vi "Create from TCP-IP.vi"(5 "Local Host":string="127.0.0.1", 7 "Local Port":i32=2222, 8 "Error In":errorcluster, 9 "Remote Port":i32=22, 10 "Remote Host":string="127.0.0.1", 11 "Session":refnum<class "Session.lvclass">) -> (0 "Error Out":errorcluster, 3 "Channel":refnum<class "Channel.lvclass">)   [LabVIEW 2018, in "Toolkit.lvlib" / "Channel.lvclass"]
uses:
  Channel.lvclass
  Session/Session.lvclass
  Session/Session.lvclass/Session.ctl
  SSH/SSH.lvclass/SSH.ctl
  Channel.lvclass/Channel.ctl
  Toolkit.lvlib
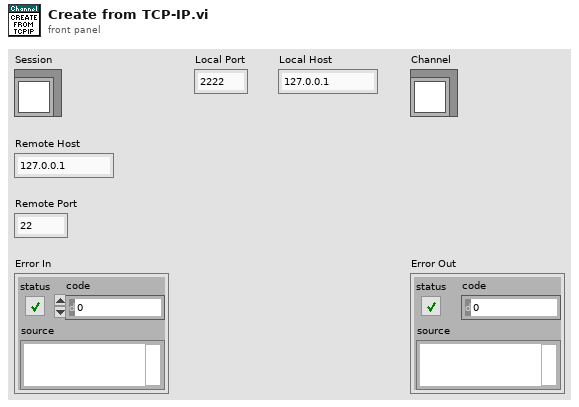
[diagram p1: front panel]
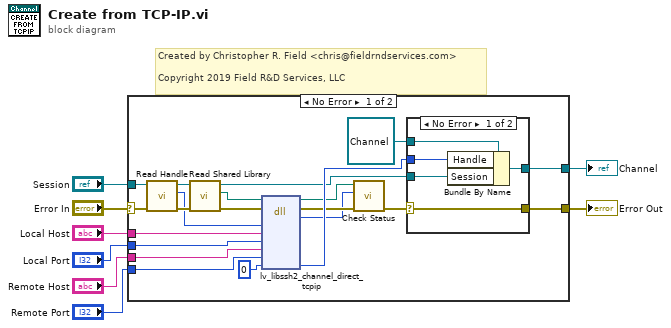
[diagram p0: block diagram]
diagram:
  # "Created by Christopher R. Field <chris@fieldrndservices.com>\n\nCopyright 2019 Field R&D Services, LLC"
  n1 = case shown="No Error" "Error In" {
    selector: "Error In" -> [w27 w37]
    tunnel: [w15 w37] -> w7
    tunnel: "Session" -> [w28 _]
    tunnel: [w29 _] -> w5
    tunnel: "Local Host" -> [w12 _]
    tunnel: "Local Port" -> [w11 _]
    tunnel: "Remote Host" -> [w10 _]
    tunnel: "Remote Port" -> [w9 _]
    frame No Error {
      n2 = call "Read Handle.vi"("Error In"=w27, "Session In"=w28) -> ("Erorr Out"=w25:errorcluster, "Handle"=w22:u64, "Session Out"=w26:refnum<class "Session.lvclass">)  [unwired: 7 in]
      n3 = call "Read Shared Library.vi"("Error In"=w25, "Session In"=w26) -> ("Erorr Out"=w24:errorcluster, "libssh2lv Shared Library"=w23:path, "Session Out"=w14:refnum<class "Session.lvclass">)  [unwired: 7 in]
      n4 = dll-call lib="libssh2lv.*" fn="lv_libssh2_channel_direct_tcpip"(path in=w23, error in=w24, "session"=w22, "host"=w12, "port"=w11, "server_host"=w10, "server_port"=w9, "handle"=u64 0) -> (path out=w17:path, error out=w19:errorcluster, "status"=w18:i32, "handle"=w20:u64)  [unwired: 6 in]
      n5 = call "Check Status.vi"("Error In"=w19, "Status"=w18, "lv-libssh2 Shared Library In"=w17) -> ("Error Out"=w16:errorcluster)  [unwired: 7 in, 1 out]
      n6 = case shown="No Error" w16 {
        selector: w16 -> [w33 w36]
        tunnel: [w30 w35] -> w29
        tunnel: w20 -> [w34 _]
        tunnel: [w33 w36] -> w15
        tunnel: w14 -> [w32 _]
        tunnel: refnum<class "Channel.lvclass"> refnum ("Toolkit.lvlib:Channel.lvclass") -> [w31 w35]
        frame No Error {
          n7 = Bundle By Name(cluster=w31, "Handle"=w34, "Session"=w32) -> (w30:refnum<class "Channel.lvclass">)
        }
        frame Error {
        }
      }
    }
    frame Error {
    }
  }
  "Error Out" <- w7
  "Channel" <- w5
